vi "String to Action.vi"(6 "Motor Labels":string[](array[string]), 7 "String":string, 8 "error in (no error)":errorcluster, 9 "Data Names&Types":string[][](array[string]), 10 "String Format":string, 11 "Action Name":string) -> (0 "error out":errorcluster, 3 "Data":string[](array[string]))   [LabVIEW 2016, in "Hardware.lvlib" / "Motions.lvlib" / "Motions.lvclass"]
uses:
  <userlib>/Common Components/Hardware/Abstract System/Motions/Motions/Motions.lvclass
panel:
  # "names"
  # "types"
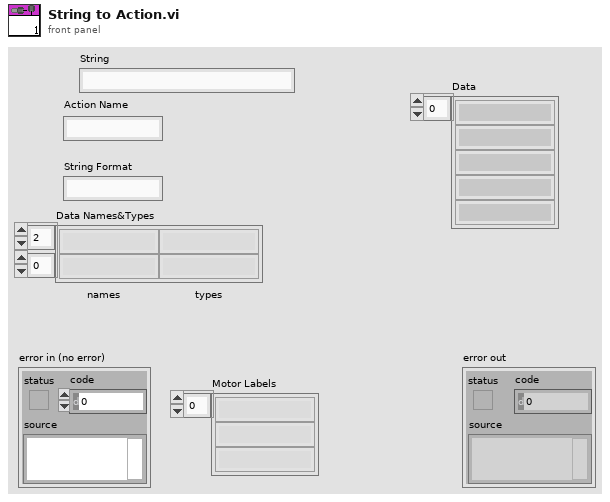
[diagram p1: front panel]
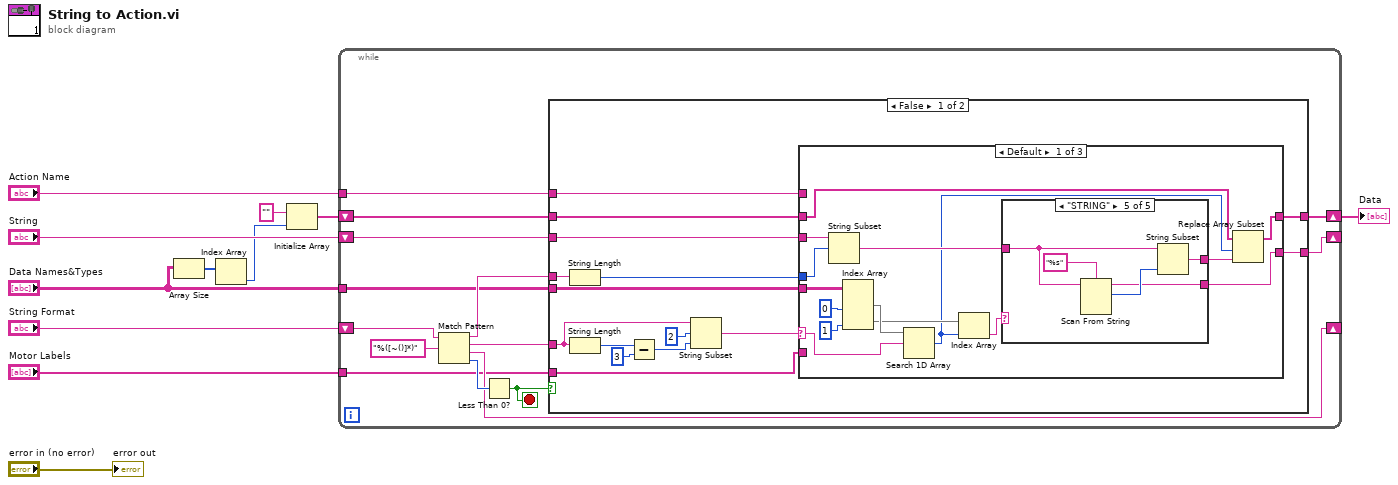
[diagram p0: block diagram]
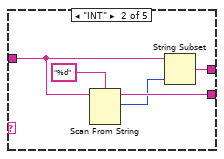
[diagram p3: hidden frame]
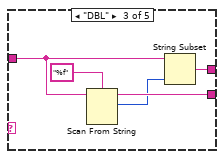
[diagram p4: hidden frame]
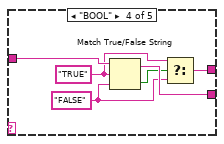
[diagram p5: hidden frame]
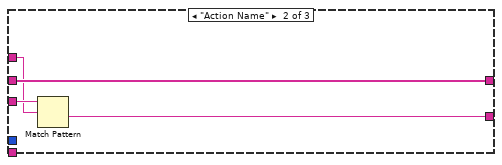
[diagram p6: hidden frame]
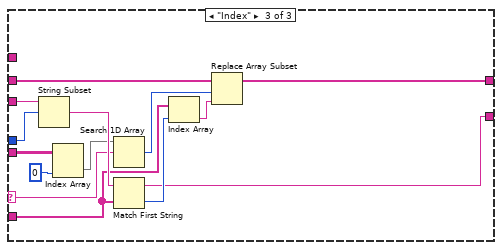
[diagram p7: hidden frame]
diagram:
  n1 = Array Size(array="Data Names&Types") -> (size(s)=w5:i32[])
  n2 = Index Array(array=w5) -> (element=w3:i32)  [unwired: 1 in]
  n3 = Initialize Array("", w3) -> (w2:string[])
  n4 = while {
    tunnel: "Action Name" -> [w20]
    shift-right: [w19] -> _
    shift-left: "String Format" -> [w25]
    tunnel: "Data Names&Types" -> [w17]
    shift-right: [w15] -> _
    shift-left: "String" -> [w16]
    tunnel: "Motor Labels" -> [w14]
    shift-right: [w12] -> w1
    shift-left: w2 -> [w13]
    stop <- w18 stop-if-true
    n5 = Match Pattern(string=w25, regular expression="%([~()]*)") -> (before substring=w22:string, match substring=w21:string, after substring=w19:string, offset past match=w23:i32)  [unwired: 1 in]
    n6 = Less Than 0?(x=w23) -> (x < 0?=w18:bool)
    n7 = case shown="False" w18 {
      tunnel: w22 -> [w30 _]
      tunnel: w21 -> [w39 _]
      tunnel: w20 -> [w34 _]
      tunnel: w17 -> [w33 _]
      tunnel: w16 -> [w32 _]
      tunnel: [w31 _] -> w15
      tunnel: w14 -> [w28 _]
      tunnel: w13 -> [w27 w96]
      tunnel: [w26 w96] -> w12
      frame False {
        n8 = String Length(string=w30) -> (length=w29:i32)
        n9 = String Length(string=w39) -> (length=w38:i32)
        n10 = Subtract(x=w38, y=3) -> (x-y=w36:i32)
        n11 = String Subset(string=w39, offset (0)=2, length (rest)=w36) -> (substring=w35:string)
        n12 = case shown="Default" w35 {
          selector: w35 -> [w55 _ w88]
          tunnel: w34 -> [_ w78 _]
          tunnel: w33 -> [w54 _ w90]
          tunnel: w32 -> [w48 w81 w95]
          tunnel: [w45 w80 w82] -> w31
          tunnel: w29 -> [w47 _ w94]
          tunnel: w28 -> [_ _ w92]
          tunnel: w27 -> [w43 w79 w86]
          tunnel: [w42 w79 w84] -> w26
          frame Default {
            n13 = String Subset(string=w48, offset (0)=w47) -> (substring=w46:string)  [unwired: 1 in]
            n14 = Index Array(array=w54, index (col) #1=0 ("disabled index (col)"), index (col) #2=1 ("index (col)")) -> (element #1=w52:string[], element #2=w50:string[])  [unwired: 2 in]
            n15 = Search 1D Array(1D array=w52, element=w55) -> (index of element=w41:i32)  [unwired: 1 in]
            n16 = Index Array(array=w50, index=w41) -> (element=w49:string)
            n17 = case shown="\"STRING\"" w49 {
              tunnel: w46 -> [w56 w59 w64 w72 w75]
              tunnel: [w56 w60 w65 w71 w74] -> w45
              tunnel: [_ w57 w62 w67 w73] -> w44
              frame Default {
              }
              frame "INT" {
                n18 = Scan From String(format string="%d", input string=w59) -> (remaining string=w60:string, offset past scan=w58:u32)  [unwired: 4 in, 1 out]
                n19 = String Subset(string=w59, length (rest)=w58) -> (substring=w57:string)  [unwired: 1 in]
              }
              frame "DBL" {
                n20 = Scan From String(format string="%f", input string=w64) -> (remaining string=w65:string, offset past scan=w63:u32)  [unwired: 4 in, 1 out]
                n21 = String Subset(string=w64, length (rest)=w63) -> (substring=w62:string)  [unwired: 1 in]
              }
              frame "BOOL" {
                w68 = "FALSE" ("false string")
                w69 = "TRUE" ("true string")
                n22 = Match True/False String(2:w68, 3:w69, 4:w72) -> (0:w70:bool, 1:w71:string)
                n23 = Select(t=w69, s=w70, f=w68) -> (s? t:f=w67:string)
              }
              frame "STRING" {
                n24 = Scan From String(format string="%s", input string=w75) -> (remaining string=w74:string, offset past scan=w76:u32)  [unwired: 4 in, 1 out]
                n25 = String Subset(string=w75, length (rest)=w76) -> (substring=w73:string)  [unwired: 1 in]
              }
            }
            n26 = Replace Array Subset(array=w43, new element=w44, index=w41) -> (w42:string[])
          }
          frame "Action Name" {
            n27 = Match Pattern(string=w81, regular expression=w78) -> (after substring=w80:string)  [unwired: 1 in, 3 out]
          }
          frame "Index" {
            n28 = String Subset(string=w95, offset (0)=w94) -> (substring=w93:string)  [unwired: 1 in]
            n29 = Index Array(array=w90, index (col)=0 ("disabled index (col)")) -> (element=w89:string[])  [unwired: 1 in]
            n30 = Search 1D Array(1D array=w89, element=w88) -> (index of element=w87:i32)  [unwired: 1 in]
            n31 = Match First String(2:w92, 3:w93) -> (0:w91:i32, 1:w82:string)
            n32 = Index Array(array=w92, index=w91) -> (element=w85:string)
            n33 = Replace Array Subset(array=w86, new element=w85, index=w87) -> (w84:string[])
          }
        }
      }
      frame True {
      }
    }
  }
  "Data" <- w1
  "error out" <- "error in (no error)"
